vi "VI Tester Menu Activation.vi"(8 "error in":errorcluster, 9 "Last Test":string, 10 "Active VI Info":T1) -> (0 "error out":errorcluster, 2 "Menu String":string)   [LabVIEW 2009]
uses:
  <vilib>/addons/_JKI Toolkits/RCF API/Right Click API.llb/Framework - Active VI Info - Cluster - __RightClickAPI.ctl
  <vilib>/addons/_JKI Toolkits/RCF API/Right Click API.llb/Framework - Selection Type - Enum - __RightClickAPI.ctl
  <userlib>/_OpenG.lib/array/array.llb/Conditional Auto-Indexing Tunnel (String)__ogtk.vi
  <userlib>/_OpenG.lib/file/file.llb/Strip Path Extension - String__ogtk.vi
  <vilib>/addons/_JKI Toolkits/RCF API/Right Click API.llb/RightClickAPI.lvlib
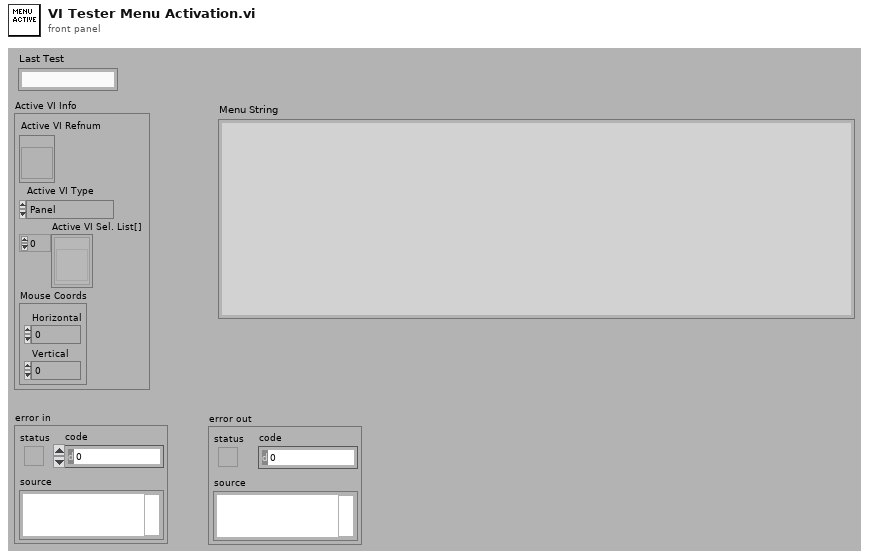
[diagram p1: front panel]
types:
  T1 = typedef "RightClickAPI.lvlib/Framework - Active VI Info - Cluster - __RightClickAPI.ctl" = cluster{"Active VI Refnum":refnum<vi>, "Active VI Type":T2, "Active VI Sel. List[]":refnum<vi>[], "Mouse Coords":cluster{"Horizontal":i32, "Vertical":i32}}
  T2 = typedef "RightClickAPI.lvlib/Framework - Selection Type - Enum - __RightClickAPI.ctl" = enum16{"Panel", "Diagram"}
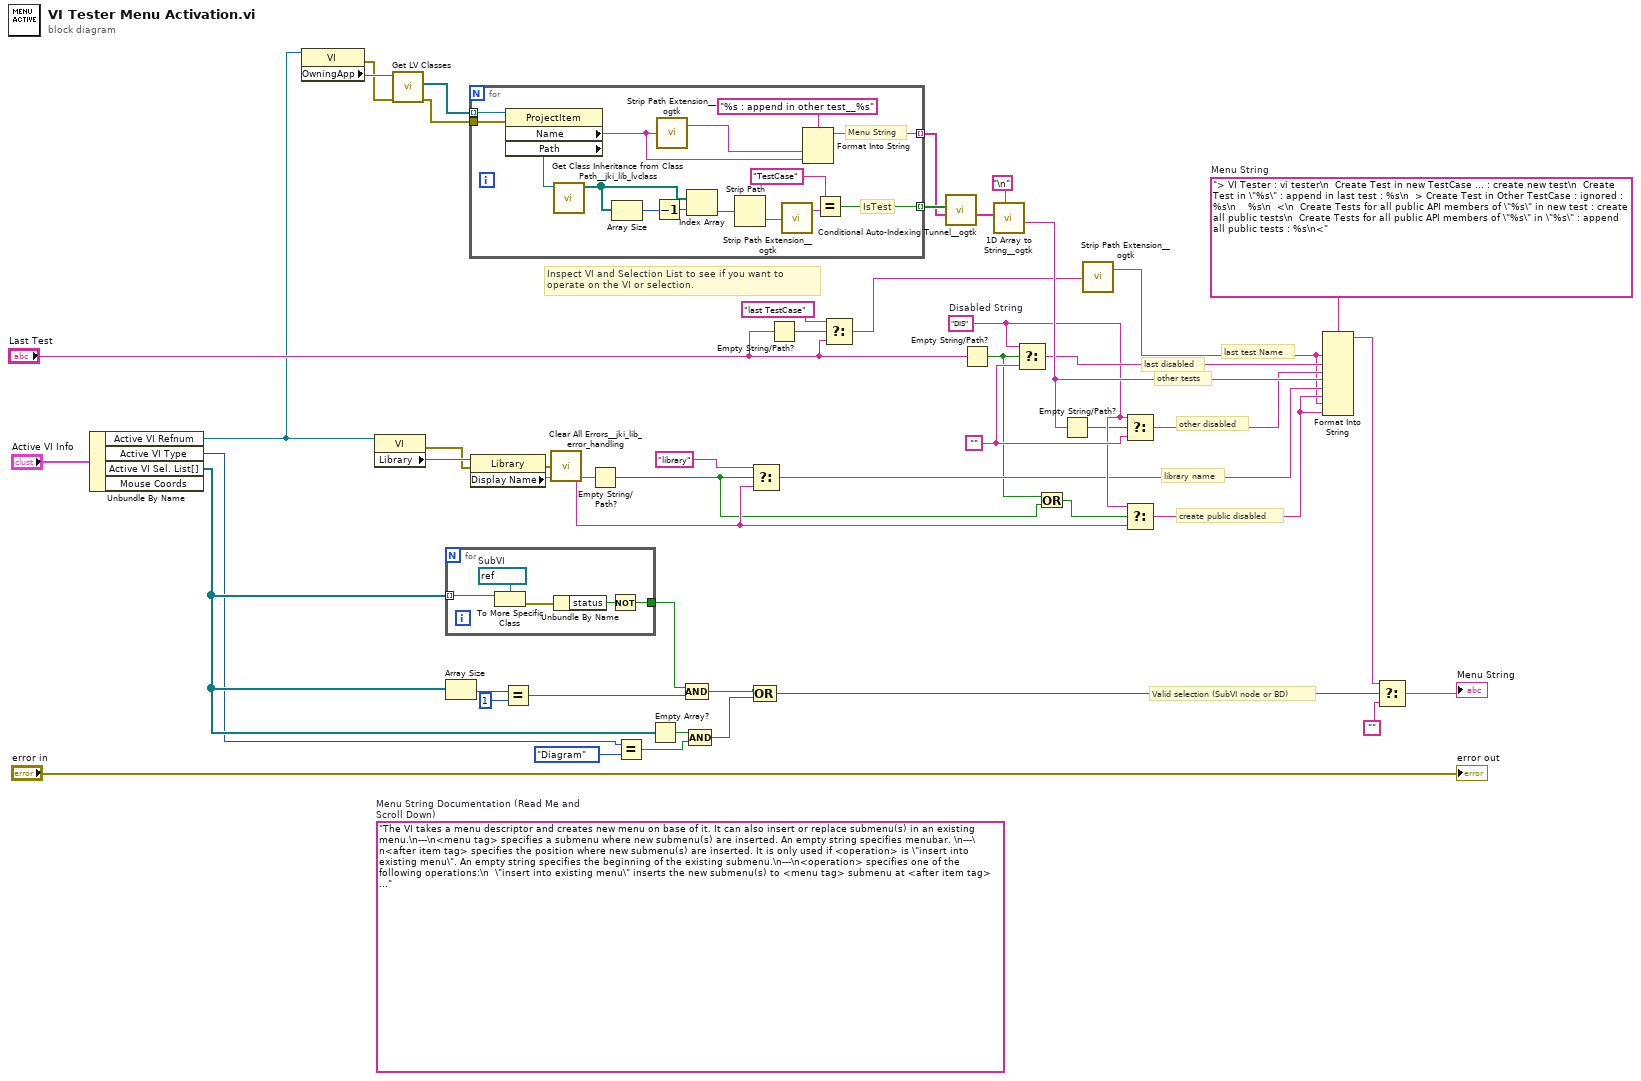
[diagram p0: block diagram]
diagram:
  w21 = ""
  w28 = "> VI Tester : vi tester\n  Create Test in new TestCase ... : create new test\n  Create Test in \"%s\" : append in last test : %s\n  > Create Test in Other TestCase : ignored : %s\n    %s\n  <\n  Create Tests for all public API members of \"%s\" in new test : create all public tests\n  Create Tests for all public API members of \"%s\" in \"%s\" : append all public tests : %s\n<"  # Menu String
  (unwired) "The VI takes a menu descriptor and creates new menu on base of it. It can also insert or replace submenu(s) in an existing menu.\n---\n<menu tag> specifies a submenu where new submenu(s) are inserted. An empty string specifies menubar. \n---\n<after item tag> specifies the position where new submenu(s) are inserted. It is only used if <operation> is \"insert into existing menu\". An empty string specifies the beginning of the existing submenu.\n---\n<operation> specifies one of the following operations:\n  \"insert into existing menu\" inserts the new submenu(s) to <menu tag> submenu at <after item tag> position.\n  \"append to existing submenu\" appends the new submenu(s) to the end of <menu tag> submenu.\n  \"replace existing menu\" replaces all the items in the <menu tag> submenu with the new submenu(s).\n---\n<menu descriptor> is a multi-line string where each line contains a menu item attributes. Empty lines and lines beginning with semicolon (;) are ignored. A line starting with a dash sign (-) forms a separator in menu. A descriptor line has the following format:\n\n  [SubMenuSign] ItemName : ItemTag [ : ItemParams [ : comments] ]\n\nSybMenuSign is optional parameter that can be either greater-than sign (>) marking the beginning of new submenu or less-than sign (<) marking the end of submenu. If a line begins with less-than sign (<), the rest of the line is ignored. You can form nested submenus providing that each '>' block is terminated with '<'.\n\nItemNames and ItenTags are respectively a name of menu item and a tag of menu item. If an item name includes a underscore sign (_), the following character is used for ALT navigation. \n\nItemParams can contain optional specificators of the menu item separated by spaces. The specificators are not case-sensitive. You can use the following specificators:\nDIS - menu item is disabled\nCHK - menu item is checked\nKEY=CHAR - specifies a shortcut keys combination. If CHAR begins with '@' sign, the shortcut is CTRL-SHIFT-CHAR; otherwise, it is CTRL-CHAR.\n\nExample:\n------------\n; File menu\n> File : file\n  _Open... : open : key=O\n  _Close... : close : key=C\n  -  ;separator\n  ; nested submenu\n  > Configuration : config\n    Parameter 1 : cfg_1 : CHK : checked\n    Parameter 2 : cfg_2 : DIS : disabled\n  <\n  -  ;separator\n  E_xit : exit : key=X\n<\n; Mode menu\n> Mode : mode\nmode 1 : mode1 : KEY=@A CHK\nmode 2 : mode2 : KEY=@B DIS\nmode 3 : mode3 : KEY=@C\n<\n"  # Menu String Documentation (Read Me and Scroll Down)
  w12 = "DIS"  # Disabled String
  # "library name"
  # "create public disabled"
  # "Valid selection (SubVI node or BD)"
  # "other tests"
  # "other disabled"
  # "last disabled"
  # "last test Name"
  # "Inspect VI and Selection List to see if you want to operate on the VI or selection."
  n1 = Unbundle By Name("Active VI Info") -> ("Active VI Refnum"=w14:refnum<vi>, "Active VI Type"=w37:T2, "Active VI Sel. List[]"=w40:refnum<vi>[])  [unwired: 1 out]
  n2 = property class="VI"(reference=w14) -> (error out=w31:errorcluster, "OwningApp"=w32:refnum<vi>)  [unwired: 1 in, 1 out]
  n3 = property class="VI"(reference=w14) -> (error out=w9:errorcluster, "Library"=w13:refnum<vi>)  [unwired: 1 in, 1 out]
  n4 = call "Get LV Classes.vi"("error in (no error)"=w31, "App reference"=w32) -> ("error out"=w30:errorcluster, "LabVIEW Classes"=w29:refnum<vi>[])  [unwired: 7 in, 1 out]
  n5 = for {
    tunnel: w40 -> [w53] mode=indexing
    tunnel: [w50] -> w42
    w49 = refnum<vi> refnum  # SubVI
    n6 = To More Specific Class(target class=w49, reference=w53) -> (error out=w52:errorcluster)  [unwired: 1 in, 1 out]
    n7 = Unbundle By Name(w52) -> ("status"=w51:bool)
    n8 = Not(x=w51) -> (.not. x?=w50:bool)
  }
  n9 = Array Size(array=w40) -> (size(s)=w44:i32)
  n10 = for {
    tunnel: w30 -> [w68]
    tunnel: w29 -> [w67] mode=indexing
    tunnel: [w66] -> w24 mode=indexing
    tunnel: [w55] -> w25 mode=indexing
    # "Menu String"
    # "IsTest"
    n11 = property class="ProjectItem"(reference=w67, error in=w68) -> ("Name"=w54:string, "Path"=w63:path)  [unwired: 2 out]
    n12 = call <vilib>:"Get Class Inheritance from Class Path__jki_lib_lvclass.vi"("lvclass file Path"=w63) -> ("Class Inheritance [ ]"=w60:path[])  [unwired: 9 in, 1 out]
    n13 = Array Size(array=w60) -> (size(s)=w62:i32)
    n14 = Decrement(x=w62) -> (x-1=w61:i32)
    n15 = call-poly <userlib>:"Strip Path Extension__ogtk.vi"("path"=w54) -> ("root"=w64:string)  [unwired: 1 out]
    n16 = Index Array(array=w60, index=w61) -> (element=w59:path)
    n17 = Strip Path(path=w59) -> (name=w58:string)  [unwired: 1 out]
    n18 = call-poly <userlib>:"Strip Path Extension__ogtk.vi"("path"=w58) -> ("root"=w57:string)  [unwired: 1 out]
    n19 = Format Into String(format string="%s : append in other test__%s", w64, w54) -> (resulting string=w66:string)  [unwired: 2 in, 1 out]
    n20 = Equal?(x="TestCase", y=w57) -> (x = y?=w55:bool)
  }
  n21 = property class="Library"(reference=w13, error in=w9) -> (error out=w8:errorcluster, "Display Name"=w10:string)  [unwired: 1 out]
  n22 = Equal?(x=w44, y=1) -> (x = y?=w41:bool)
  n23 = call <vilib>:"Clear All Errors__jki_lib_error_handling.vi"("error in"=w8) -> ()  [unwired: 4 in, 1 out]
  n24 = Empty String/Path?(string/path=w10) -> (empty?=w5:bool)
  n25 = Equal?(x=w37, y=Framework_-_Selection_Type_-_Enum_-___RightClickAPI."Diagram" ("Active VI Type")) -> (x = y?=w36:bool)
  n26 = Empty Array?(array=w40) -> (empty?=w39:bool)
  n27 = Compound Arithmetic op=AND(w42, w41) -> (w34:bool)
  n28 = Compound Arithmetic op=AND(w39, w36) -> (w35:bool)
  n29 = Select(t="library", s=w5, f=w10) -> (s? t:f=w7:string)
  n30 = Compound Arithmetic op=OR(w34, w35) -> (w33:bool)
  n31 = Empty String/Path?(string/path="Last Test") -> (empty?=w18:bool)
  n32 = Select(t="last TestCase", s=w18, f="Last Test") -> (s? t:f=w15:string)
  n33 = call-poly <userlib>:"Conditional Auto-Indexing Tunnel__ogtk.vi"("Array in"=w24, "Elements to keep"=w25) -> ("Filtered Array out"=w23:string[])  [unwired: 5 in]
  n34 = Empty String/Path?(string/path="Last Test") -> (empty?=w6:bool)
  n35 = call <userlib>:"1D Array to String__ogtk.vi"("delimiter (Tab)"="\n", "Array of Strings"=w23) -> ("delimited string"=w22:string)  [unwired: 9 in]
  n36 = Select(t=w12, s=w6, f=w21) -> (s? t:f=w19:string)
  n37 = Or(x=w6, y=w5) -> (x .or. y?=w4:bool)
  n38 = Empty String/Path?(string/path=w22) -> (empty?=w1:bool)
  n39 = call-poly <userlib>:"Strip Path Extension__ogtk.vi"("path"=w15) -> ("root"=w2:string)  [unwired: 1 out]
  n40 = Select(t=w12, s=w1, f=w21) -> (s? t:f=w20:string)
  n41 = Select(t=w12, s=w4, f=w10) -> (s? t:f=w3:string)
  n42 = Format Into String(format string=w28, w2, w19, w20, w22, w7, w3, w2, w3) -> (resulting string=w27:string)  [unwired: 2 in, 1 out]
  n43 = Select(t=w27, s=w33, f="") -> (s? t:f=→"Menu String":string)
  "error out" <- "error in"
